vi "subSeguridad.vi"(1 "z":bool, 2 "y":bool, 3 "x":bool) -> (0 ".not. (x .and. y)?":bool)   [LabVIEW 2020]
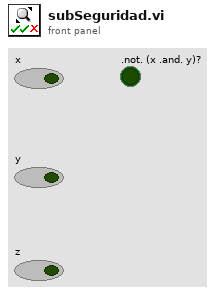
[diagram p1: front panel]
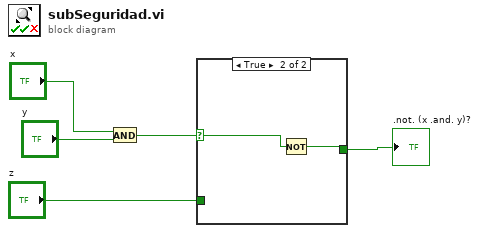
[diagram p0: block diagram]
diagram:
  n1 = And(x="x", y="y") -> (x .and. y?=w2:bool)
  n2 = case shown="True" w2 {
    selector: w2 -> [_ w8]
    tunnel: "z" -> [w6 _]
    tunnel: [w6 w7] -> w1
    frame False {
    }
    frame True {
      n3 = Not(x=w8) -> (.not. x?=w7:bool)
    }
  }
  ".not. (x .and. y)?" <- w1
